vi "Set Delay Generator.vi"(8 "error in (no error)":errorcluster, 9 "typ":i32, 10 "address":i16, 11 "board":i32) -> (0 "error out":errorcluster, 3 "function return":u32)   [LabVIEW 2014, in "atmcd32d.lvlib"]
doc: "unsigned int WINAPI SetDelayGenerator(int board, short address, int typ);"
uses:
  atmcd32d.lvlib
  atmcd32d.dll
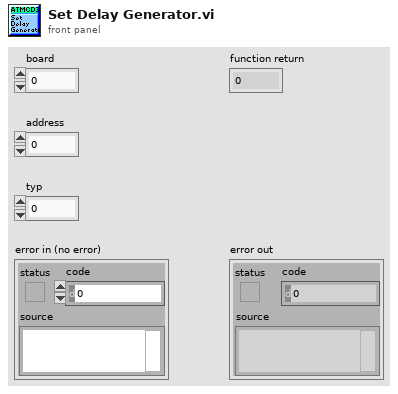
[diagram p1: front panel]
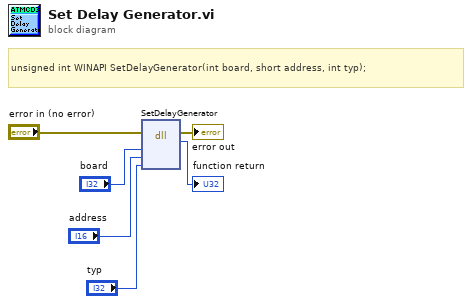
[diagram p0: block diagram]
diagram:
  # "unsigned int WINAPI SetDelayGenerator(int board, short address, int typ);"
  n1 = dll-call lib="C:/Users/Bakir/Documents/Lambda2-Testing/lib/Andorlib/atmcd32d.*" fn="SetDelayGenerator"(error in="error in (no error)", "board"="board", "address"="address", "typ"="typ") -> (error out=→"error out":errorcluster, →"function return":u32)  [unwired: 5 in, 1 out]
